vi "Arguments to Array of Variants.vi"(8 "error in (no error)":errorcluster, 9 "input string":string, 10 "Inputs":variant, 11 "input type":variant) -> (0 "error out":errorcluster, 2 "Array":variant[](array[variant]))   [LabVIEW 2021, in "smo.lvlib" / "SMOFacade.lvclass"]
uses:
  SMOFacade.lvclass
  SMOFacade.lvclass/SMOFacade.ctl
  smo.lvlib
  <vilib>/Utility/VariantDataType/VariantType.lvlib
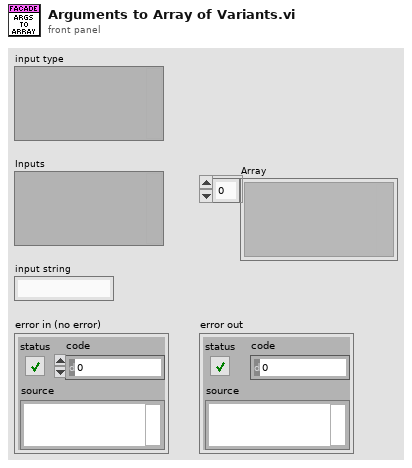
[diagram p1: front panel]
types:
  T1 = typedef "VariantType.lvlib/Type.ctl" = enum8{"Invalid Type", "Void", "I8", "I16", "I32", "I64", "U8", "U16", "U32", "U64", "Single Float", "Double Float", "Extended Float", "Single Complex", "Double Complex", "Extended Complex", "Enum U8", "Enum U16", "Enum U32", "Enum U64", "Single Float With Unit", "Double Float With Unit", "Extended Float With Unit", "Single Complex with Unit", "Double Complex with Unit", "Extended Complex with Unit", "Boolean", "String", "Path", "Picture", "Tag", "Array", "Cluster", "Variant", "LV Variant", "Waveform", "Timestamp", "Digital Waveform", "Digital Data", "ExpressData", "Refnum", "External Data", "VI", "Poly VI", "LabVIEW Class Instance", "Fixed Point"}
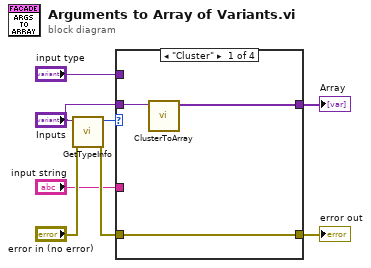
[diagram p0: block diagram]
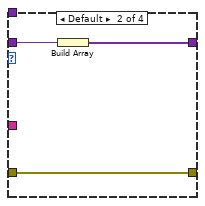
[diagram p2: hidden frame]
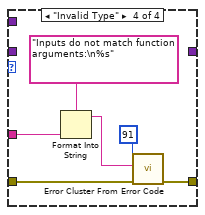
[diagram p4: hidden frame]
diagram:
  n1 = call <vilib>:"GetTypeInfo.vi"("error in (no error)"="error in (no error)", "Variant"="Inputs") -> ("error out"=w5:errorcluster, "Type Enum"=w3:T1)  [unwired: 5 in, 3 out]
  n2 = case shown="\"Cluster\"" w3 {
    tunnel: [w11 w12 w15 w20] -> w1
    tunnel: w5 -> [w11 w12 w15 w21]
    tunnel: "input string" -> [_ _ _ w18]
    tunnel: "Inputs" -> [w10 w14 _ _]
    tunnel: [w9 w13 _ _] -> w7
    tunnel: "input type" -> [_ _ _ _]
    frame "Cluster" {
      n3 = call "ClusterToArray.vi"("Cluster"=w10) -> ("Array"=w9:variant[])  [unwired: 10 in]
    }
    frame Default {
      n4 = Build Array(w14) -> (w13:variant[])
    }
    frame "Void" {
    }
    frame "Invalid Type" {
      n5 = Format Into String(format string="Inputs do not match function arguments:\n%s" ("error message (\"\")"), w18) -> (resulting string=w16:string)  [unwired: 2 in, 1 out]
      n6 = call <vilib>:"Error Cluster From Error Code.vi"("error in (no error)"=w21, "error message (\"\")"=w16, "error code (0)"=91) -> ("error out"=w20:errorcluster)  [unwired: 6 in]
    }
  }
  "Array" <- w7
  "error out" <- w1
